vi "Abort.vi"(8 "error in (no error)":errorcluster, 11 "SMO":refnum<class "SMO.lvclass">) -> (0 "error out":errorcluster, 3 "SMO out":refnum<class "SMO.lvclass">)   [LabVIEW 2021, in "smo.lvlib" / "SMO.lvclass"]
doc: "---------------------------------------------------------------\nJKI State Machine Objects™\nhttp://jki.net/state-machine-objects/\nCopyright (C) 2005-2015, JKI <info@jki.net>\nALL RIGHTS RESERVED"
uses:
  SMO.lvclass
  SMO.lvclass/SMO.ctl
  ReftoDVR--SMO.vi
panel:
  # "For instructions on how to use the JKI State Machine Objects, examples and video tutorials, visit:\nhttp://jki.net/state-machine-objects/\n\nJKI State Machine Objects™\nhttp://jki.net/state-machine-objects/\nCopyright (C) 2005-2015, JKI <info@jki.net>\nALL RIGHTS RESERVED"
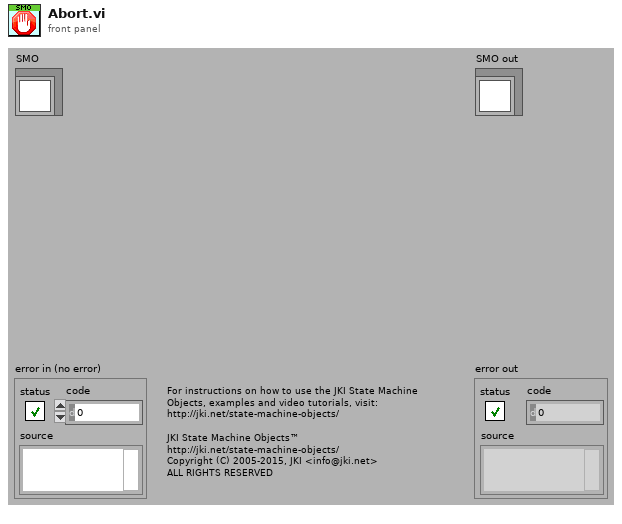
[diagram p1: front panel]
types:
  T1 = typedef "smo.lvlib/SMO.lvclass/Protected Events.ctl" = cluster{"StopProcesses":refnum<user-event>, "AbortProcesses":refnum<user-event>, "Config Changed":refnum<user-event>, "Dependency":refnum<user-event>}
  T2 = typedef "smo.lvlib/SMO.lvclass/RegisteredProcessData--Cluster.ctl" = cluster{"Name":string, "Static VI Ref":refnum<vi>, "Running":bool, "NotifierRef":u32}
  T3 = enum32{"Bad", "Idle", "Run top level", "Running"}
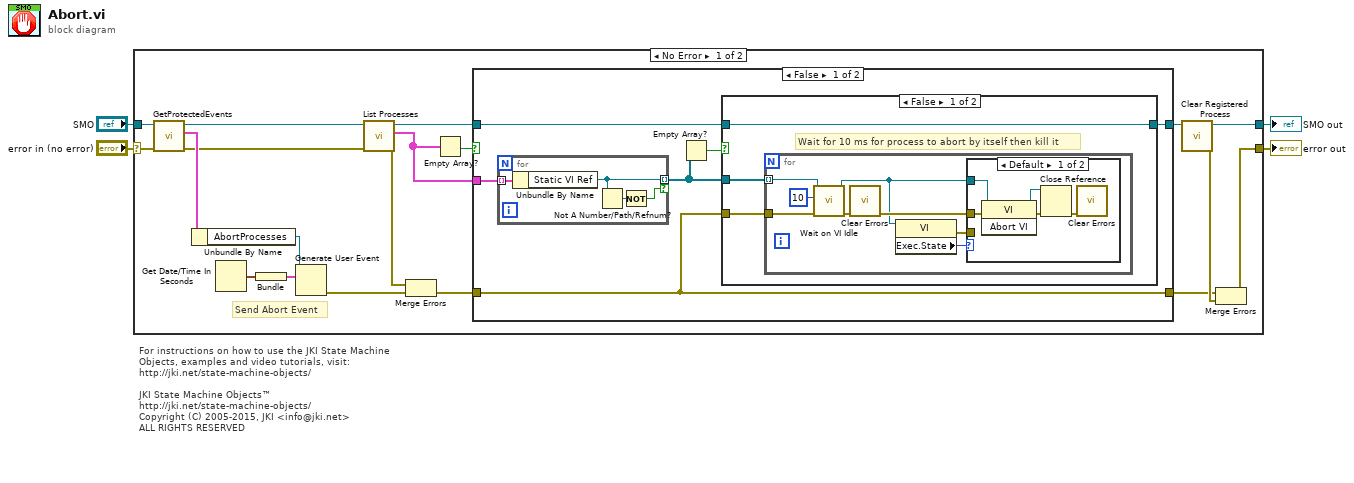
[diagram p0: block diagram]
diagram:
  # "For instructions on how to use the JKI State Machine Objects, examples and video tutorials, visit:\nhttp://jki.net/state-machine-objects/\n\nJKI State Machine Objects™\nhttp://jki.net/state-machine-objects/\nCopyright (C) 2005-2015, JKI <info@jki.net>\nALL RIGHTS RESERVED"
  n1 = case shown="No Error" "error in (no error)" {
    selector: "error in (no error)" -> [w9 w54]
    tunnel: [w21 w54] -> w3
    tunnel: [w20 w53] -> w1
    tunnel: "SMO" -> [w11 w53]
    frame No Error {
      # "Send Abort Event"
      n2 = call "GetProtectedEvents.vi"("error in (no error)"=w9, "SMO"=w11) -> ("error out"=w8:errorcluster, "SMO Protected Events"=w15:T1, "SMO out"=w10:refnum<class "SMO.lvclass">)  [unwired: 7 in]
      n3 = Unbundle By Name(w15) -> ("AbortProcesses"=w14:refnum<user-event>)
      n4 = Get Date/Time In Seconds() -> (seconds since 1Jan1904=w22:timestamp)
      n5 = Bundle("seconds since 1Jan1904"=w22) -> (w23:cluster{"seconds since 1Jan1904":timestamp})  [unwired: 1 in]
      n6 = Generate User Event(user event=w14, event data cluster=w23) -> (error out=w6:errorcluster)  [unwired: 2 in, 1 out]
      n7 = call "List Processes.vi"("error in (no error)"=w8, "SMO"=w10) -> ("error out"=w7:errorcluster, "Registered Processes"=w13:T2[], "SMO out"=w12:refnum<class "SMO.lvclass">)  [unwired: 7 in]
      n8 = Merge Errors(w7, w6) -> (w5:errorcluster)
      n9 = Empty Array?(array=w13) -> (empty?=w18:bool)
      n10 = case shown="False" w18 {
        tunnel: w13 -> [w29 _]
        tunnel: w5 -> [w28 w51]
        tunnel: w12 -> [w26 w52]
        tunnel: [w25 w52] -> w17
        tunnel: [w28 w51] -> w16
        frame False {
          n11 = for {
            tunnel: w29 -> [w48] mode=indexing
            tunnel: [w47] -> w27 mode=indexing if=w49
            n12 = Unbundle By Name(w48) -> ("Static VI Ref"=w47:refnum<vi>)
            n13 = Not A Number/Path/Refnum?(number/path/refnum=w47) -> (NaN/Path/Refnum?=w50:bool)
            n14 = Not(x=w50) -> (.not. x?=w49:bool)
          }
          n15 = Empty Array?(array=w27) -> (empty?=w24:bool)
          n16 = case shown="False" w24 {
            tunnel: w28 -> [w32 _]
            tunnel: w27 -> [w31 _]
            tunnel: w26 -> [w30 w46]
            tunnel: [w30 w46] -> w25
            frame False {
              # "Wait for 10 ms for process to abort by itself then kill it"
              n17 = for {
                tunnel: w32 -> [w40]
                tunnel: w31 -> [w36] mode=indexing
                n18 = call "Wait on VI Idle.vi"("error in (no error)"=w40, "ms Timout (100ms)"=u32 10, "VI to Wait on"=w36) -> ("error out"=w38:errorcluster, "VI to Wait on dup"=w35:refnum<vi>)  [unwired: 6 in, 1 out]
                n19 = call <vilib>:"Clear Errors.vi"("error in (no error)"=w38) -> ("error out"=w37:errorcluster)  [unwired: 5 in, 1 out]
                n20 = property class="VI"(reference=w35) -> (error out=w33:errorcluster, "Exec.State"=w34:T3)  [unwired: 1 in, 1 out]
                n21 = case shown="Default" w34 {
                  tunnel: w37 -> [w45 _]
                  tunnel: w35 -> [w41 _]
                  tunnel: w33 -> [_ _]
                  frame Default {
                    n22 = invoke class="VI" method="Abort VI"(reference=w41, error in=w45) -> (reference out=w42:refnum<vi>, error out=w44:errorcluster)  [unwired: 1 in, 1 out]
                    n23 = Close Reference(reference=w42, error in (no error)=w44) -> (error out=w43:errorcluster)
                    n24 = call <vilib>:"Clear Errors.vi"("error in (no error)"=w43) -> ()  [unwired: 5 in, 2 out]
                  }
                  frame "Bad", "Idle" {
                  }
                }
              }
            }
            frame True {
            }
          }
        }
        frame True {
        }
      }
      n25 = call "Clear Registered Process.vi"("SMO"=w17) -> ("error out"=w19:errorcluster, "SMO out"=w20:refnum<class "SMO.lvclass">)  [unwired: 9 in]
      n26 = Merge Errors(w16, w19) -> (w21:errorcluster)
    }
    frame Error {
    }
  }
  "error out" <- w3
  "SMO out" <- w1
